vi "Construct.vi"(8 "error in (no error)":errorcluster, 9 "Owning VI":path, 10 "LangFile ref":refnum<data-value>, 11 "GObject in":refnum<class "GObject.lvclass">) -> (0 "error out":errorcluster, 3 "GObject out":refnum<class "GObject.lvclass">)   [LabVIEW 2013, in "SET Project Data.lvlib" / "GObject.lvclass"]
uses:
  GObject.lvclass
  Resource Data Class/Resource Data.lvclass
  GObject.lvclass/GObject.ctl
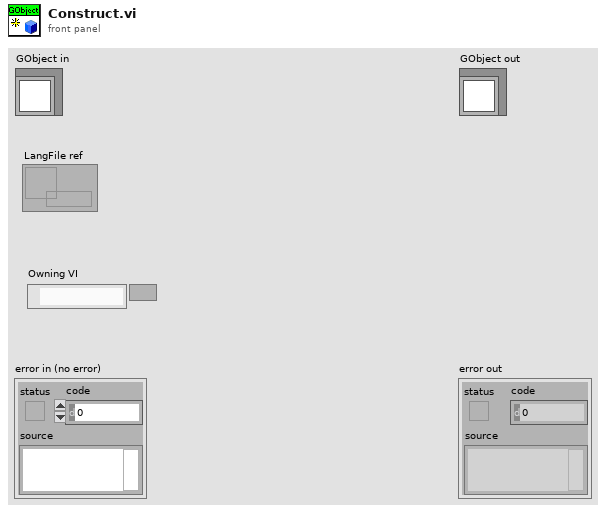
[diagram p1: front panel]
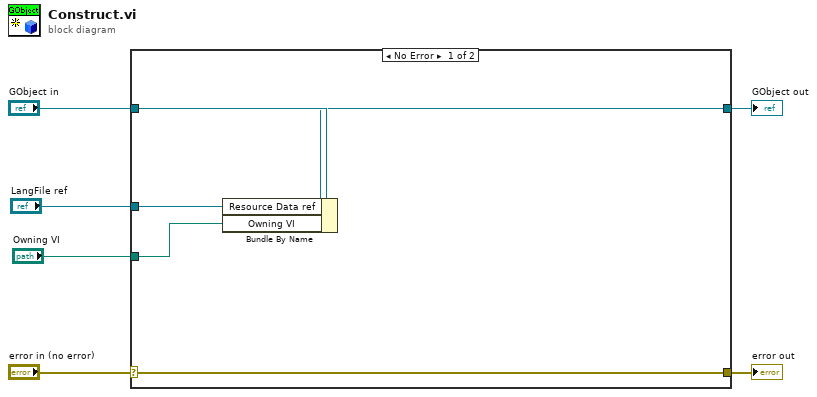
[diagram p0: block diagram]
diagram:
  n1 = case shown="No Error" "error in (no error)" {
    selector: "error in (no error)" -> [w11 w13]
    tunnel: [w11 w13] -> w5
    tunnel: [w9 w12] -> w3
    tunnel: "GObject in" -> [w10 w12]
    tunnel: "LangFile ref" -> [w8 _]
    tunnel: "Owning VI" -> [w7 _]
    frame No Error {
      n2 = Bundle By Name(cluster=w10, "Resource Data ref"=w8, "Owning VI"=w7) -> (w9:refnum<class "GObject.lvclass">)
    }
    frame Error {
    }
  }
  "error out" <- w5
  "GObject out" <- w3
